vi "Read XML HW Configuration File_Parse Channels_Extract Fields From RawData.vi"(0 "rawData":string[](array[string])) -> (1 "label":u32, 2 "Word.InitialValue":u32, 3 "SDIValue":u8 format="%.0b")   [LabVIEW 2020, in "Ballard Arinc-429 System Explorer.lvlib"]
uses:
  Ballard Arinc-429 System Explorer.lvlib
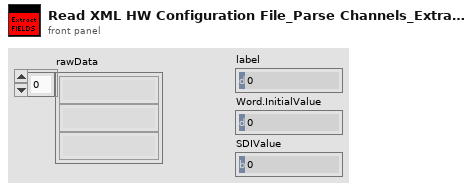
[diagram p1: front panel]
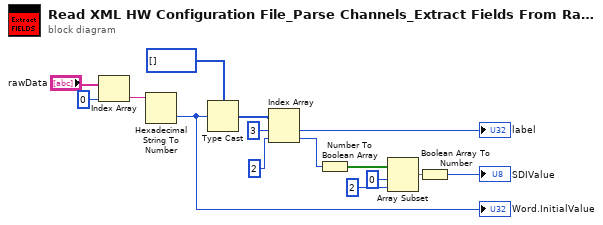
[diagram p0: block diagram]
diagram:
  n1 = Index Array(array="rawData", index=0) -> (element=w13:string)
  n2 = Hexadecimal String To Number(string=w13) -> (number=w11:u32)  [unwired: 2 in, 1 out]
  "Word.InitialValue" <- w11
  n3 = Type Cast(type=u8[] [], x=w11) -> (*(type *) &x=w10:u8[])
  n4 = Index Array(array=w10, index #1=3 ("index"), index #2=2 ("index")) -> (element #1=→"label":u8, element #2=w6:u8)
  n5 = Number To Boolean Array(number=w6) -> (Boolean array=w3:bool[])
  n6 = Array Subset(array=w3, index=0, length=2) -> (w2:bool[])
  n7 = Boolean Array To Number(Boolean array=w2) -> (number=→"SDIValue":u8)
